vi "Test of Get Path Loss.vi"() -> ()   [LabVIEW 2020, in "PathControl.lvclass"]
uses:
  PathControl.lvclass
  Measurements Specific Paths.ctl
  Paths.ctl
panel:
  out "XY Graph":cluster{dbl[], dbl[]}[](graph)
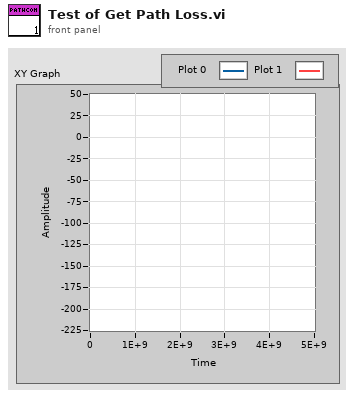
[diagram p1: front panel]
types:
  T1 = typedef "PathControl.lvclass/Measurements Specific Paths.ctl" = enum16{"No calibration", "Harmonics", "IMD", "S Parameter", "AM-AM", "MCCW-ACLR", "DC", "LCR", "Power Meter GUI", "RF Power"}
  T2 = typedef "PathControl.lvclass/Paths.ctl" = enum16{"SigGen 1 -> DUT", "SigGen 2 -> DUT", "SigGen 1 -> PM 1", "SigGen 1 -> PM 2", "DUT -> SA", "DUT -> PM 2", "VSG -> DUT", "SigGen 2 -> PM 1", "SigGen 2 -> PM 2"}
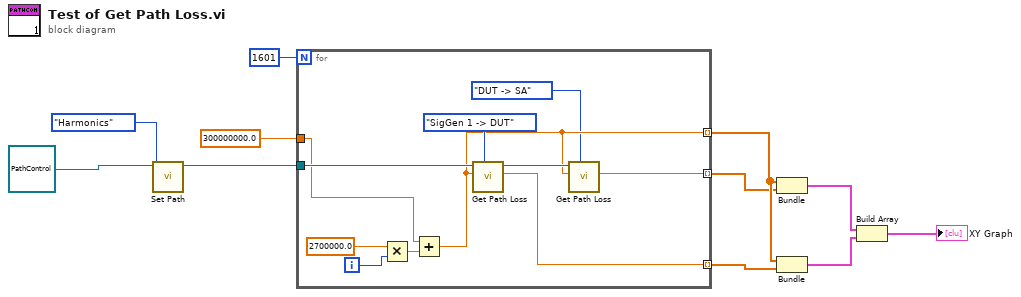
[diagram p0: block diagram]
diagram:
  n1 = call "Set Path.vi"("Measurement specfic paths"=Measurements_Specific_Paths."Harmonics", "PathControl in"=refnum<class "PathControl.lvclass"> refnum ("PathControl.lvclass")) -> ("PathControl out"=w9:refnum<class "PathControl.lvclass">)  [unwired: 8 in, 1 out]
  n2 = for {
    N: 1601 -> [_]
    tunnel: w9 -> [w22]
    tunnel: 300000000.0 -> [w16]
    tunnel: [w15] -> w5 mode=indexing
    tunnel: [w14] -> w6 mode=indexing
    tunnel: [w13] -> w4 mode=indexing
    i -> [w19]
    n3 = Multiply(x=2700000.0, y=w19) -> (x*y=w17:dbl)
    n4 = Add(x=w16, y=w17) -> (x+y=w15:dbl)
    n5 = call "Get Path Loss.vi"("Path"=Paths."SigGen 1 -> DUT", "Frequency [Hz]"=w15, "PathControl in"=w22) -> ("Insertion Loss (dB)"=w14:dbl, "PathControl out"=w20:refnum<class "PathControl.lvclass">)  [unwired: 5 in, 2 out]
    n6 = call "Get Path Loss.vi"("Path"=Paths."DUT -> SA", "Frequency [Hz]"=w15, "PathControl in"=w20) -> ("Insertion Loss (dB)"=w13:dbl)  [unwired: 5 in, 3 out]
  }
  n7 = Bundle(w5, w4) -> (w3:cluster{dbl[], dbl[]})  [unwired: 1 in]
  n8 = Bundle(w5, w6) -> (w2:cluster{dbl[], dbl[]})  [unwired: 1 in]
  n9 = Build Array(w3, w2) -> (→"XY Graph":cluster{dbl[], dbl[]}[])
